vi "Is Data Ready.vi"(8 "error in (no error)":errorcluster, 11 "Ni-Scope Digitizer in":refnum<class "Ni-Scope Digitizer.lvclass">) -> (0 "error out":errorcluster, 1 "Data ready":bool, 2 "Availiable Samples":u32, 3 "Ni-Scope Digitizer out":refnum<class "Ni-Scope Digitizer.lvclass">)   [LabVIEW 2015, in "Ni-Scope Digitizer.lvclass"]
uses:
  Ni-Scope Digitizer.lvclass
  Instruments/Pulse Driver/Pulse Driver.lvclass/Pulse Driver.ctl
  Ni-Scope Digitizer.lvclass/Ni-Scope Digitizer.ctl
  Instruments/Pulse Driver/Read Samples per read.vi
  Instruments/Pulse Driver/Read Samples per channel.vi
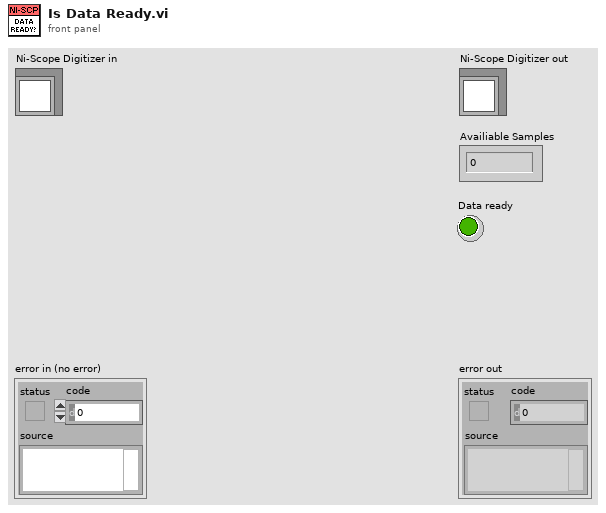
[diagram p1: front panel]
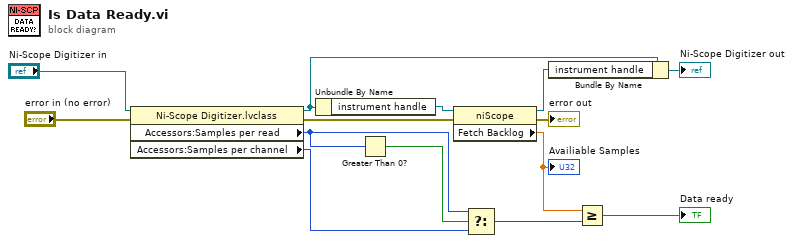
[diagram p0: block diagram]
diagram:
  n1 = property class="Ni-Scope Digitizer.lvclass"(reference="Ni-Scope Digitizer in", error in="error in (no error)") -> (reference out=w8:refnum<class "Ni-Scope Digitizer.lvclass">, error out=w1:errorcluster, "Accessors:Samples per read"=w5:i32, "Accessors:Samples per channel"=w4:i32)
  n2 = Unbundle By Name(w8) -> ("instrument handle"=w14:refnum<k15>)
  n3 = Greater Than 0?(x=w5) -> (x > 0?=w6:bool)
  n4 = property class="niScope"(reference=w14, error in=w1) -> (reference out=w13:refnum<k15>, error out=→"error out":errorcluster, "Fetch Backlog"=w10:dbl)
  "Availiable Samples" <- w10
  n5 = Select(t=w5, s=w6, f=w4) -> (s? t:f=w3:i32)
  n6 = Bundle By Name(cluster=w8, "instrument handle"=w13) -> (→"Ni-Scope Digitizer out":refnum<class "Ni-Scope Digitizer.lvclass">)
  n7 = Greater Or Equal?(x=w10, y=w3) -> (x >= y?=→"Data ready":bool)
